vi "Discrete Filter.vi"   [LabVIEW 2020, in "NI_AdvCtrl_discrete linear.lvlib"]
doc: "LabVIEW no longer supports this VI. You can obtain similar functionality by installing the LabVIEW Simulation Module.\n\nFilters the set of input data using the direct form IIR filter specified by Reverse Coefficients and Forward Coefficients."
uses:
  <vilib>/addons/control/advanced/NI_AdvCtrl_discrete linear.lvlib
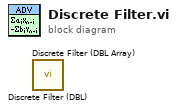
[diagram p0: block diagram]
diagram:
  n1 = call <vilib>:"Discrete Filter (DBL).vi"() -> ()  [unwired: 5 in, 1 out]
  n2 = call <vilib>:"Discrete Filter (DBL Array).vi"() -> ()  [unwired: 5 in, 1 out]
